vi "ReadForLoop.vi"(2 "reference":refnum<vi>) -> (1 "ForLoop":T7)   [LabVIEW 2013]
uses:
  <vilib>/Utility/miscctls.llb/LVBoundsTypeDef.ctl
  <vilib>/Utility/miscctls.llb/LVRectTypeDef.ctl
  <vilib>/Utility/miscctls.llb/LVPositionTypeDef.ctl
  <vilib>/Utility/miscctls.llb/LVBreakpointStatusEnum.ctl
  <vilib>/picture/picture.llb/imagedata.ctl
  <vilib>/Utility/miscctls.llb/LVParallelSchedulesEnum.ctl
panel:
  out "error out":errorcluster
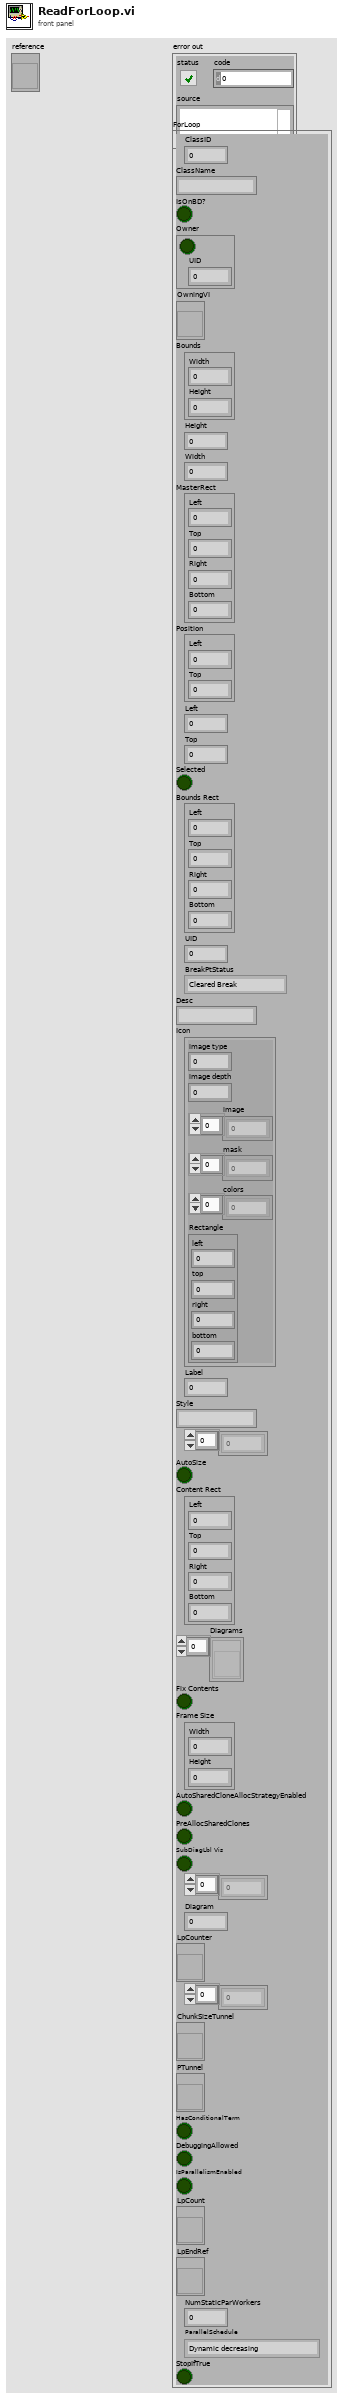
[diagram p1: front panel]
types:
  T1 = typedef "LVBoundsTypeDef.ctl" = cluster{"Width":u32, "Height":u32}
  T2 = typedef "LVRectTypeDef.ctl" = cluster{"Left":i16, "Top":i16, "Right":i16, "Bottom":i16}
  T3 = typedef "LVPositionTypeDef.ctl" = cluster{"Left":i32, "Top":i32}
  T4 = typedef "LVBreakpointStatusEnum.ctl" = enum8{"Cleared Break", "Enabled Break", "Disabled Break"}
  T5 = typedef "imagedata.ctl" = cluster{"image type":i32, "image depth":i32, "image":u8[], "mask":u8[], "colors":u32[], "Rectangle":cluster{"left":i16, "top":i16, "right":i16, "bottom":i16}}
  T6 = typedef "LVParallelSchedulesEnum.ctl" = enum8{"Dynamic decreasing", "Dynamic fixed size", "Static block", "Static block-cyclic"}
  T7 = cluster{"ClassID":u32, "ClassName":string, "IsOnBD?":bool, "Owner":cluster{bool, "UID":i32}, "OwningVI":refnum<vi>, "Bounds":T1, "Height":u32, "Width":u32, "MasterRect":T2, "Position":T3, "Left":i32, "Top":i32, "Selected":bool, "Bounds Rect":T2, "UID":i32, "BreakPtStatus":T4, "Desc":string, "Icon":T5, "Label":i32, "Style":string, "Terms[]":i32[], "AutoSize":bool, "Content Rect":T2, "Diagrams":refnum<vi>[], "Fix Contents":bool, "Frame Size":T1, "AutoSharedCloneAllocStrategyEnabled":bool, "PreAllocSharedClones":bool, "SubDiagLbl Vis":bool, "Tunnels[]":i32[], "Diagram":i32, "LpCounter":refnum<vi>, "ShiftRegs[]":i32[], "ChunkSizeTunnel":refnum<vi>, "PTunnel":refnum<vi>, "HasConditionalTerm":bool, "DebuggingAllowed":bool, "IsParallelismEnabled":bool, "LpCount":refnum<vi>, "LpEndRef":refnum<vi>, "NumStaticParWorkers":i32, "ParallelSchedule":T6, "StopIfTrue":bool}
  T8 = cluster{"ClassID":u32, "ClassName":string, "IsOnBD?":bool, "Cluster":cluster{bool, "UID":i32}, "OwningVI":refnum<vi>, "Bounds":T1, "Height":u32, "Width":u32, "MasterRect":T2, "Position":T3, "Left":i32, "Top":i32, "Selected":bool, "Bounds Rect":T2, "UID":i32, "BreakPtStatus":T4, "Desc":string, "Icon":T5, "UID":i32, "Style":string, i32[], "AutoSize":bool, "Content Rect":T2, "Diagrams":refnum<vi>[], "Fix Contents":bool, "Frame Size":T1, "AutoSharedCloneAllocStrategyEnabled":bool, "PreAllocSharedClones":bool, "SubDiagLbl Vis":bool, i32[], "UID":i32, "LpCounter":refnum<vi>, i32[], "ChunkSizeTunnel":refnum<vi>, "PTunnel":refnum<vi>, "HasConditionalTerm":bool, "DebuggingAllowed":bool, "IsParallelismEnabled":bool, "LpCount":refnum<vi>, "LpEndRef":refnum<vi>, "NumStaticParWorkers":i32, "ParallelSchedule":T6, "StopIfTrue":bool}
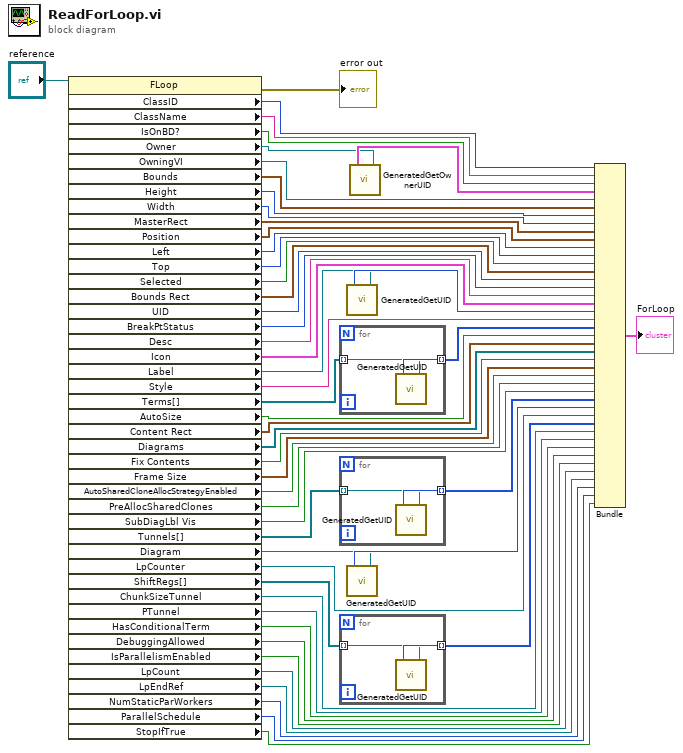
[diagram p0: block diagram]
diagram:
  n1 = property class="FLoop"(reference="reference") -> (error out=→"error out":errorcluster, "ClassID"=w50:u32, "ClassName"=w49:string, "IsOnBD?"=w48:bool, "Owner"=w46:refnum<vi>, "OwningVI"=w45:refnum<vi>, "Bounds"=w44:T1, "Height"=w43:u32, "Width"=w42:u32, "MasterRect"=w41:T2, "Position"=w40:T3, "Left"=w39:i32, "Top"=w38:i32, "Selected"=w37:bool, "Bounds Rect"=w36:T2, "UID"=w35:i32, "BreakPtStatus"=w34:T4, "Desc"=w33:string, "Icon"=w32:T5, "Label"=w30:refnum<vi>, "Style"=w29:string, "Terms[]"=w27:refnum<vi>[], "AutoSize"=w26:bool, "Content Rect"=w25:T2, "Diagrams"=w24:refnum<vi>[], "Fix Contents"=w23:bool, "Frame Size"=w22:T1, "AutoSharedCloneAllocStrategyEnabled"=w21:bool, "PreAllocSharedClones"=w20:bool, "SubDiagLbl Vis"=w19:bool, "Tunnels[]"=w17:refnum<vi>[], "Diagram"=w15:refnum<vi>, "LpCounter"=w14:refnum<vi>, "ShiftRegs[]"=w12:refnum<vi>[], "ChunkSizeTunnel"=w11:refnum<vi>, "PTunnel"=w10:refnum<vi>, "HasConditionalTerm"=w9:bool, "DebuggingAllowed"=w8:bool, "IsParallelismEnabled"=w7:bool, "LpCount"=w6:refnum<vi>, "LpEndRef"=w5:refnum<vi>, "NumStaticParWorkers"=w4:i32, "ParallelSchedule"=w3:T6, "StopIfTrue"=w2:bool)  [unwired: 1 in, 1 out]
  n2 = for {
    tunnel: [w54] -> w28 mode=indexing
    tunnel: w27 -> [w53] mode=indexing
    n3 = call "GeneratedGetUID.vi"("Text in"=w53) -> ("UID"=w54:i32)
  }
  n4 = for {
    tunnel: [w56] -> w18 mode=indexing
    tunnel: w17 -> [w55] mode=indexing
    n5 = call "GeneratedGetUID.vi"("Text in"=w55) -> ("UID"=w56:i32)
  }
  n6 = for {
    tunnel: [w58] -> w13 mode=indexing
    tunnel: w12 -> [w57] mode=indexing
    n7 = call "GeneratedGetUID.vi"("Text in"=w57) -> ("UID"=w58:i32)
  }
  n8 = call "GeneratedGetUID.vi"("Text in"=w30) -> ("UID"=w31:i32)
  n9 = call "GeneratedGetUID.vi"("Text in"=w15) -> ("UID"=w16:i32)
  n10 = call "GeneratedGetOwnerUID.vi"("Generic in"=w46) -> ("Cluster"=w47:cluster{bool, "UID":i32})
  n11 = Bundle("ClassID"=w50, "ClassName"=w49, "IsOnBD?"=w48, "Cluster"=w47, "OwningVI"=w45, "Bounds"=w44, "Height"=w43, "Width"=w42, "MasterRect"=w41, "Position"=w40, "Left"=w39, "Top"=w38, "Selected"=w37, "Bounds Rect"=w36, "UID"=w35, "BreakPtStatus"=w34, "Desc"=w33, "Icon"=w32, "UID"=w31, "Style"=w29, w28, "AutoSize"=w26, "Content Rect"=w25, "Diagrams"=w24, "Fix Contents"=w23, "Frame Size"=w22, "AutoSharedCloneAllocStrategyEnabled"=w21, "PreAllocSharedClones"=w20, "SubDiagLbl Vis"=w19, w18, "UID"=w16, "LpCounter"=w14, w13, "ChunkSizeTunnel"=w11, "PTunnel"=w10, "HasConditionalTerm"=w9, "DebuggingAllowed"=w8, "IsParallelismEnabled"=w7, "LpCount"=w6, "LpEndRef"=w5, "NumStaticParWorkers"=w4, "ParallelSchedule"=w3, "StopIfTrue"=w2) -> (→"ForLoop":T8)  [unwired: 1 in]
